vi "set_controls_enabled_state.vi"(8 "error in (no error)":errorcluster, 9 "status":T1(ring), 10 "control references":refnum<vi>[](array[refnum]), 11 "ScanModeMG091111IntrinsicImaging in":refnum<class "ImagingModeMG091111IntrinsicImaging.lvclass">) -> (0 "error out":errorcluster, 3 "ScanModeMG091111IntrinsicImaging out":refnum<class "ImagingModeMG091111IntrinsicImaging.lvclass">)   [LabVIEW 2010, in "ImagingModeMG091111IntrinsicImaging.lvclass"]
uses:
  ImagingModeMG091111IntrinsicImaging.lvclass
  ImagingModeDL091001Scaffold/ImagingModeDL091001Scaffold/ImagingModeDL091001Scaffold.lvclass
  ImagingModeMG091111IntrinsicImaging.lvclass/ImagingModeMG091111IntrinsicImaging.ctl
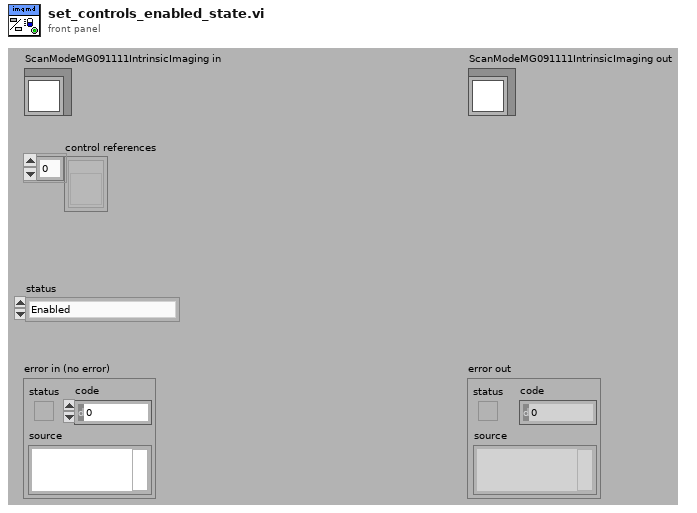
[diagram p1: front panel]
types:
  T1 = enum8{"Enabled", "Disabled", "Disabled and Grayed Out"}
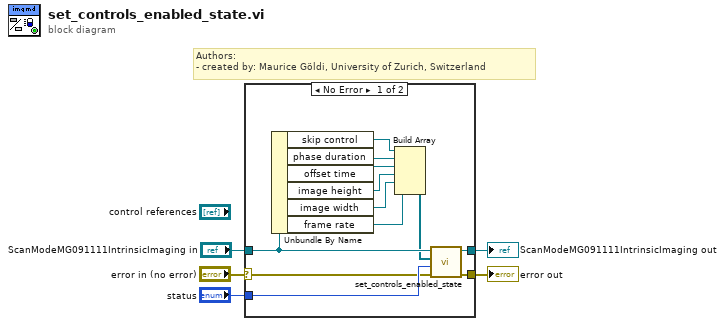
[diagram p0: block diagram]
diagram:
  # "Authors: \n- created by: Maurice Göldi, University of Zurich, Switzerland"
  n1 = case shown="No Error" "error in (no error)" {
    selector: "error in (no error)" -> [w14 w19]
    tunnel: [w17 w19] -> w5
    tunnel: [w16 w18] -> w4
    tunnel: "status" -> [w15 _]
    tunnel: "ScanModeMG091111IntrinsicImaging in" -> [w13 w18]
    frame No Error {
      n2 = Unbundle By Name(w13) -> ("skip control"=w12:refnum<vi>, "phase duration"=w11:refnum<vi>, "offset time"=w10:refnum<vi>, "image height"=w9:refnum<vi>, "image width"=w8:refnum<vi>, "frame rate"=w6:refnum<vi>)
      n3 = Build Array(w12, w11, w10, w9, w8, w6) -> (w7:refnum<vi>[])
      n4 = call-parent "set_controls_enabled_state.vi"("error in (no error)"=w14, "status"=w15, "control references"=w7, "GenericPlugin in"=w13) -> ("error out"=w17:errorcluster, "GenericPlugin out"=w16:refnum<class "ImagingModeMG091111IntrinsicImaging.lvclass">)  [unwired: 6 in]
    }
    frame Error {
    }
  }
  "error out" <- w5
  "ScanModeMG091111IntrinsicImaging out" <- w4
